vi "Format Waveform Name.vi"(1 "Waveform File Name":string) -> (0 "Waveform Name":string)   [LabVIEW 2019, in "SG.lvlib"]
doc: "Formats the waveform name in order to avoid any errors when used in a script or downloaded to the generator."
uses:
  SG.lvlib
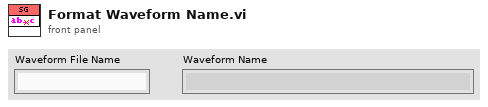
[diagram p1: front panel]
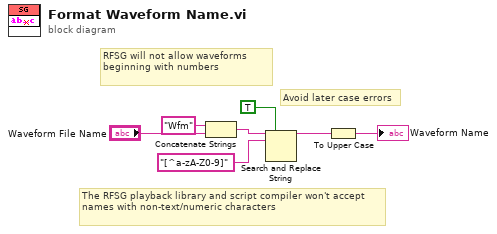
[diagram p0: block diagram]
diagram:
  # "Avoid later case errors"
  # "RFSG will not allow waveforms beginning with numbers"
  # "The RFSG playback library and script compiler won't accept names with non-text/numeric characters"
  n1 = Concatenate Strings("Wfm" ("string"), "Waveform File Name") -> (w3:string)
  n2 = Search and Replace String(replace all?=TRUE ("replace all? (F)"), input string=w3, search string="[^a-zA-Z0-9]") -> (result string=w4:string)  [unwired: 5 in, 3 out]
  n3 = To Upper Case(1:w4) -> (0:→"Waveform Name":string)
